vi "CLD3 FGV Timer no pause solution.vi"(8 "Error In":errorcluster, 10 "Time Target (s)":dbl=4.0, 11 "Timer Mode":T1) -> (0 "Error Out":errorcluster, 2 "Has Time Elapsed":bool, 3 "Elapsed Time (s.ss)":dbl)   [LabVIEW 2018]
doc: "CLD 3 Exercise"
uses:
  CLD3 FGV Mode.ctl
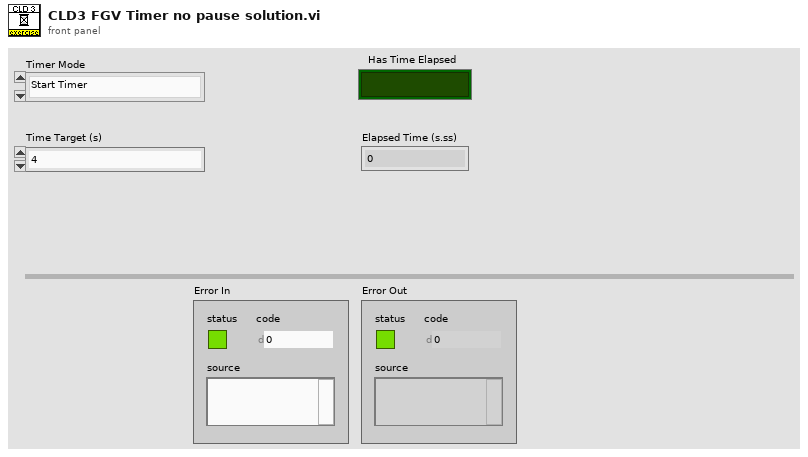
[diagram p1: front panel]
types:
  T1 = typedef "CLD3 FGV Mode.ctl" = enum16{"Start Timer", "Read Time", "Pause", "Resume"}
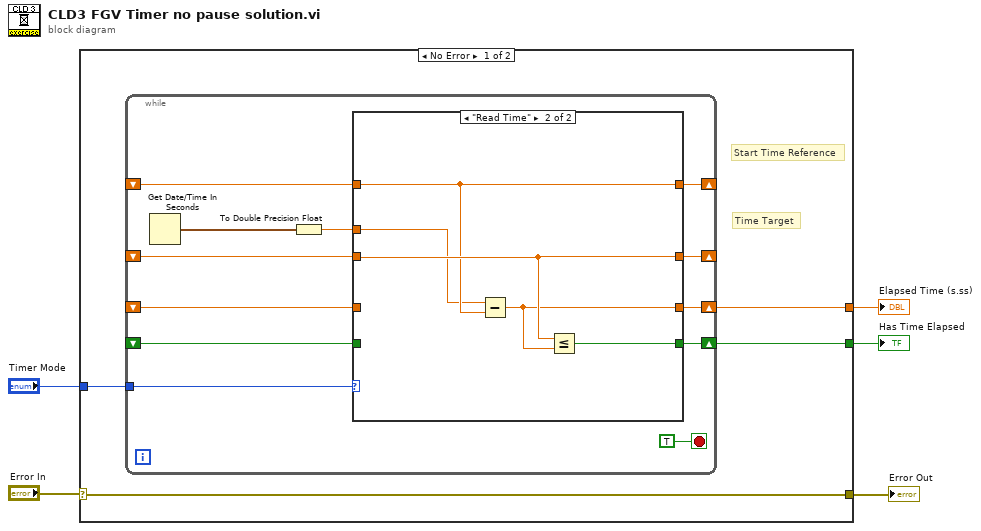
[diagram p0: block diagram]
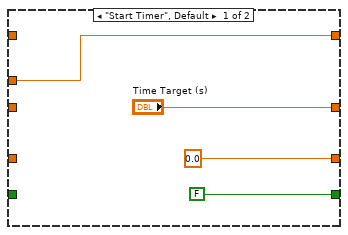
[diagram p2: hidden frame]
diagram:
  n1 = case shown="No Error" "Error In" {
    selector: "Error In" -> [w6 w31]
    tunnel: "Timer Mode" -> [w9 _]
    tunnel: [w8 _] -> w4
    tunnel: [w7 _] -> w3
    tunnel: [w6 w31] -> w1
    frame No Error {
      # "Time Target"
      # "Start Time Reference"
      n2 = while {
        tunnel: w9 -> [w21]
        shift-right: [w20] -> _
        shift-left: _ -> [w16]
        shift-right: [w18] -> _
        shift-left: _ -> [w15]
        shift-right: [w17] -> w8
        shift-left: _ -> [w13]
        shift-right: [w14] -> w7
        shift-left: _ -> [w10]
        stop <- TRUE stop-if-true
        n3 = Get Date/Time In Seconds() -> (seconds since 1Jan1904=w12:timestamp)
        n4 = To Double Precision Float(number=w12) -> (double precision float=w11:dbl)
        n5 = case shown="\"Read Time\"" w21 {
          tunnel: [w22 w27] -> w20
          tunnel: ["Time Target (s)" w30] -> w18
          tunnel: [0.0 ("Time Target (s)") w29] -> w17
          tunnel: w16 -> [_ w27]
          tunnel: w15 -> [_ w30]
          tunnel: [FALSE w28] -> w14
          tunnel: w13 -> [_ _]
          tunnel: w11 -> [w22 w26]
          tunnel: w10 -> [_ _]
          frame "Start Timer", Default {
          }
          frame "Read Time" {
            n6 = Subtract(x=w26, y=w27) -> (x-y=w29:dbl)
            n7 = Less Or Equal?(x=w30, y=w29) -> (x <= y?=w28:bool)
          }
        }
      }
    }
    frame Error {
    }
  }
  "Error Out" <- w1
  "Elapsed Time (s.ss)" <- w4
  "Has Time Elapsed" <- w3
